vi "Wait for UEGO Calibration Completion.vi"(8 "error in":errorcluster, 10 "UEGO Present?":bool, 11 "FPGA Ref in":refnum<k20>) -> (0 "error out":errorcluster)   [LabVIEW 2014, in "SLSC configuration Engine.lvlib"]
uses:
  SLSC configuration Engine.lvlib
  <vilib>/NI/LVFPGA Adv Session Resources/OpenByNameSubVI.vi
  Shared/Constants.vi
  <vilib>/rvi/interface/common/dynamic/niFpgaEscapeDelimiterAndNull.vi
  <vilib>/Utility/error.llb/Error Cluster From Error Code.vi
  <vilib>/rvi/errors/niLvFpgaAdjustHostInterfaceError.vi
  <vilib>/FPGAPlugInAG/Dynamic/niLvFpga_Close_Dynamic.vi
  <vilib>/NI/LVFPGA Adv Session Resources/OpenByName.xnode
  <vilib>/rvi/interface/nirviReadWriteControl/nirviReadWriteControl.xnode
  <vilib>/rvi/interface/nirviCloseFPGA/nirviCloseFPGA.xnode
  Shared/SLSC configuration Shared.lvlib
  NiFpgaLv.dll
  <vilib>/rvi/interface/Simulation/niFpgaSimulationCallBeginRW.vi
  <vilib>/NI/LVFPGA Adv Session Resources/LVFPGAAdvSessionResources.lvlib
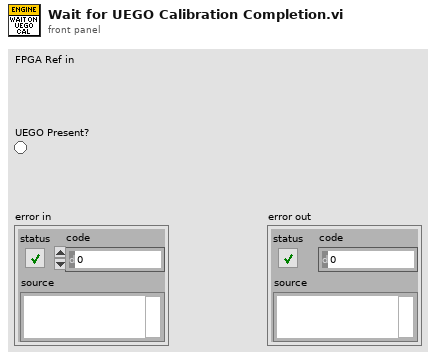
[diagram p1: front panel]
types:
  T1 = cluster{"Name":string, "Depth":u32, "Write? (Deprecated:Use Implementation)":bool, "Physical Channel":u32, "Base Address":u32, "Data Width":u32, "Data Type":enum32{"Boolean", "I8", "I16", "I32", "I64", "U8", "U16", "U32", "U64", "FXP", "CustomControl", "SGL"}, "FXP Properties":variant, "Write Window Address":u32, "Implementation":enum16{"niFpgaTargetToHost", "niFpgaHostToTarget", "niFpgaPeerToPeerWriter", "niFpgaPeerToPeerReader", "niCoreTargetToHost", "niCoreHostToTarget"}, "Control Set":u32}[]
  T2 = cluster{"Name":string, "type":variant, "indicator?":bool}[]
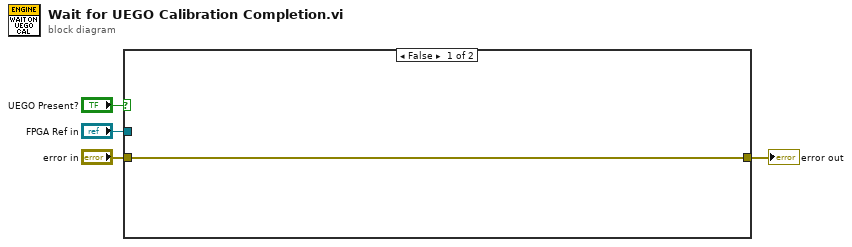
[diagram p0: block diagram]
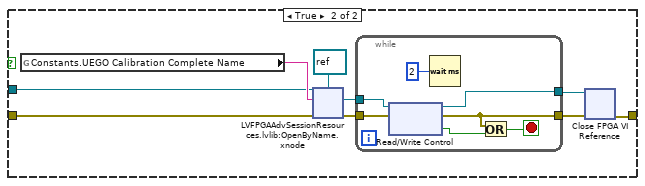
[diagram p2: hidden frame]
diagram:
  n1 = case shown="False" "UEGO Present?" {
    tunnel: "error in" -> [w5 w10]
    tunnel: [w5 w6] -> w2
    tunnel: "FPGA Ref in" -> [_ w9]
    frame False {
    }
    frame True {
      n2 = global read "Constants.vi" "Constants.UEGO Calibration Complete Name"() -> (w12:string)
      n3 = xnode "LVFPGAAdvSessionResources.lvlib:OpenByName.xnode"("FPGA VI Reference in"=w9, "Resource name in"=w12, "Single resource reference type in"=refnum<k20> refnum, "Error in"=w10) -> ("Single resource reference out"=w13:refnum<k20>, "Error out"=w14:errorcluster)  [unwired: 1 out]
      n4 = while {
        tunnel: w14 -> [w21]
        tunnel: w13 -> [w20]
        tunnel: [w17] -> w8
        tunnel: [w15] -> w7
        stop <- w16 stop-if-true
        n5 = xnode "Read/Write Control"("FPGA VI Reference In"=w20, "error in"=w21) -> ("FPGA VI Reference Out"=w15:refnum<k20>, "error out"=w17:errorcluster, "Value"=w18:bool)
        n6 = Wait (ms)(milliseconds to wait=u32 2) -> ()  [unwired: 1 out]
        n7 = Or(x=w17, y=w18) -> (x .or. y?=w16:bool)
      }
      n8 = xnode "Close FPGA VI Reference"("FPGA VI Reference In"=w7, "error in"=w8) -> ("error out"=w6:errorcluster)
    }
  }
  "error out" <- w2
